vi "Simple Serial.vi"() -> ()   [LabVIEW 2018]
doc: "This example performs a serial port write and a serial port read. The parameters set for the serial port must match the parameters of the connected instrument or device. The VISA Configure Serial Port VI sets the configuration parameters. The front panel displays the controls used to configure the basic parameters, such as baud rate, data bits, and parity. The VI passes the VISA resource name to other VIs that perform operations on that VISA resource. The VISA Write function sends a command to the serial device and the VISA Read function returns data based on the command. The VISA Close function then closes the reference to the serial device. It is important to close the reference; otherwise, further communication through that port might not be possible."
uses:
  <vilib>/Instr/_visa.llb/VISA Configure Serial Port (Instr).vi
  <vilib>/Utility/file.llb/Write Delimited Spreadsheet (string).vi
panel:
  in  "ok":bool
  out "File Path Control":path
  in  "Select Sensor":bool[](array[boolean])
  out "Sensor In Graph":dbl
  in  "stop":bool
  out "chart":T1(graph)
  in  "?":string[][](table)
  in  "Serial Settings":T2={"Number of sen"=0.0, "Baud rate"=9600, "Separator"="", "COM"="COM1"} {"Baud rate" items=["75"=75, "110"=110, "134"=134, "150"=150, "300"=300, "600"=600, "1200"=1200, "1800"=1800, "2400"=2400, "4800"=4800, "7200"=7200, "9600"=9600, "14400"=14400, "19200"=19200, "28800"=28800, "38400"=38400, "56000"=56000, "57600"=57600, "115200"=115200, "128000"=128000, "230400"=230400]}
  in  "Clear":bool
  out "working sensor indexes 2":i32[](array[numeric])
  out "Counter":dbl
  out "working sensor index":dbl[](array[numeric])
  out "working sensor":dbl[](array[numeric])
  out "output array":dbl[](array[numeric])
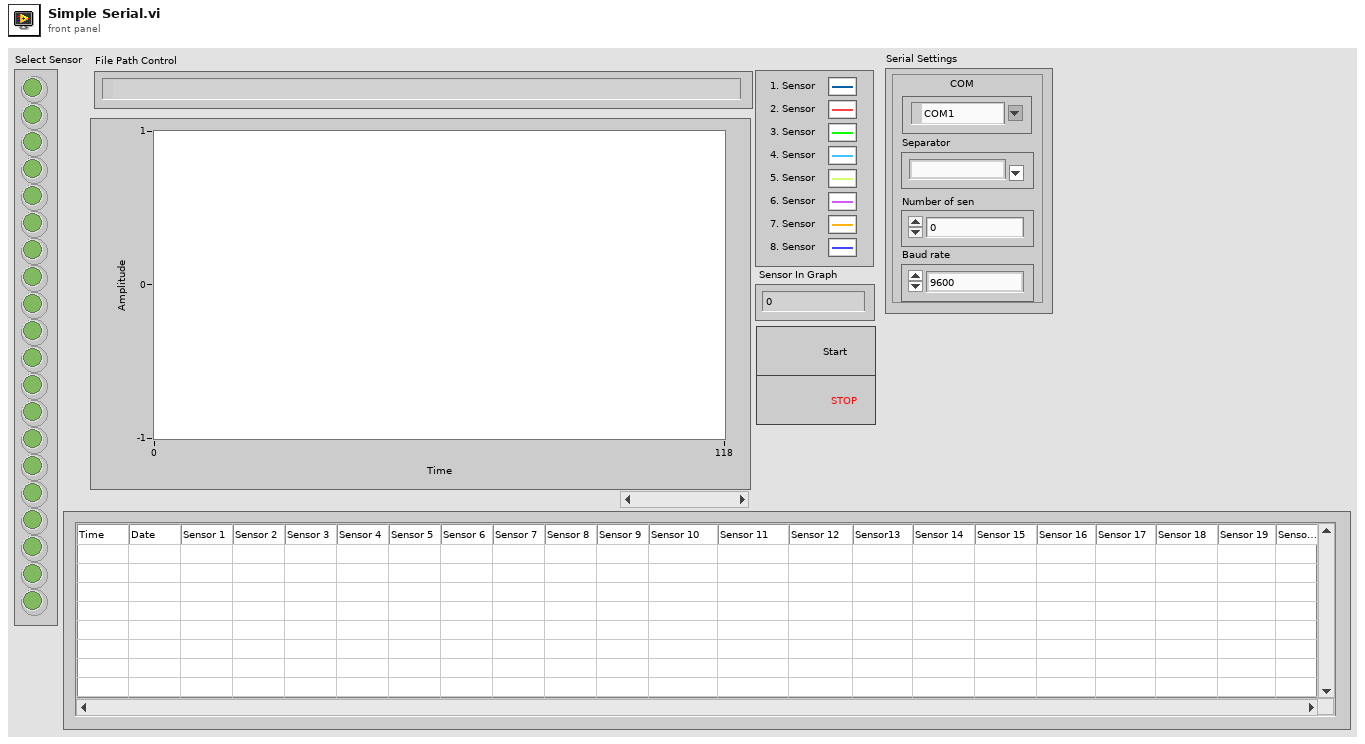
[diagram p1: front panel]
types:
  T1 = cluster{"element":dbl, "element":dbl, "element":dbl, "element":dbl, "element":dbl, "element":dbl, "element":dbl, "element":dbl}
  T2 = cluster{"Number of sen":dbl, "Baud rate":u32, "Separator":string, "COM":refnum<visa-resource-name>}
  T3 = cluster{"element":dbl, "element":dbl, "element":dbl, "element":dbl, "element":dbl, "element":dbl, "element":dbl, "element":dbl}[]
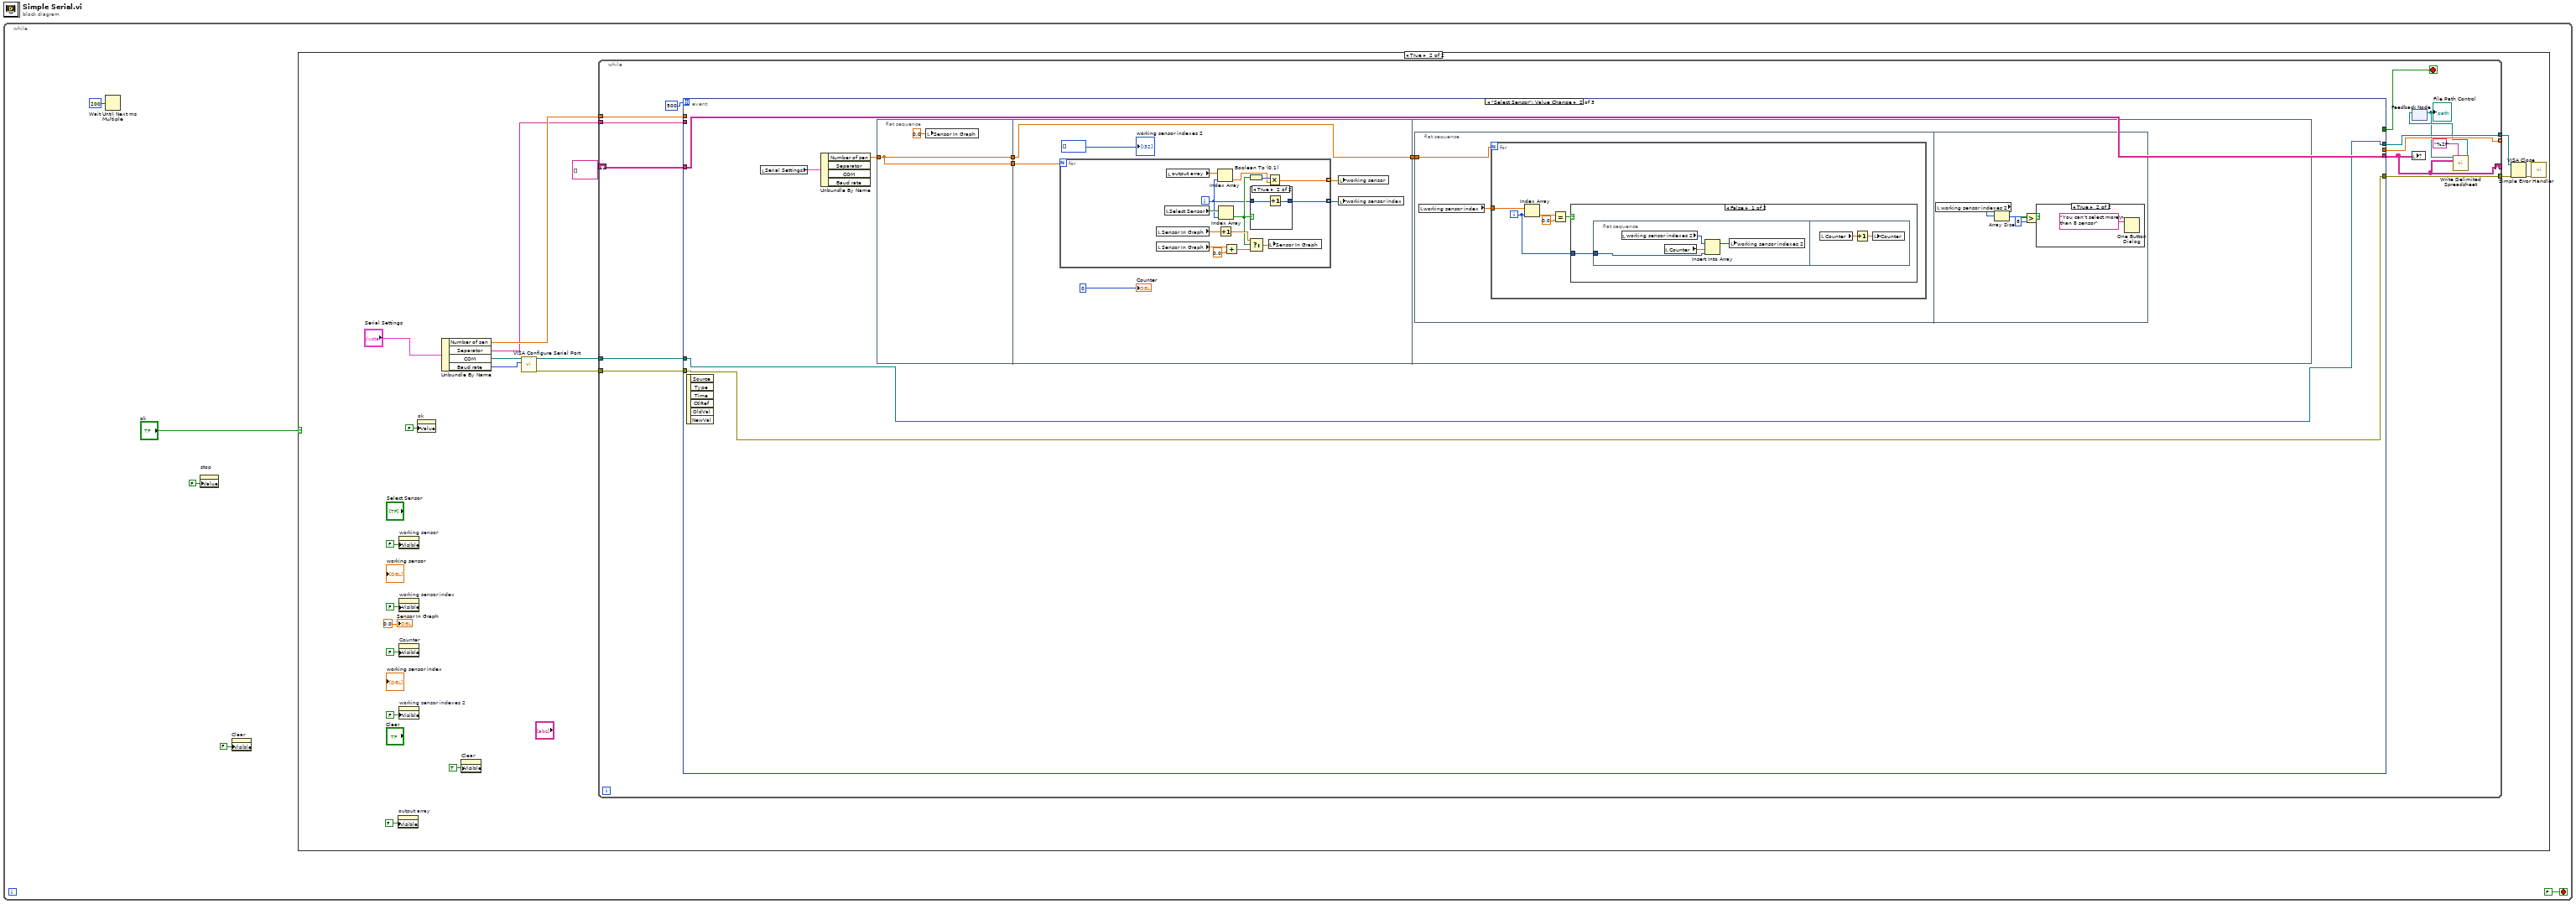
[diagram p0: block diagram]
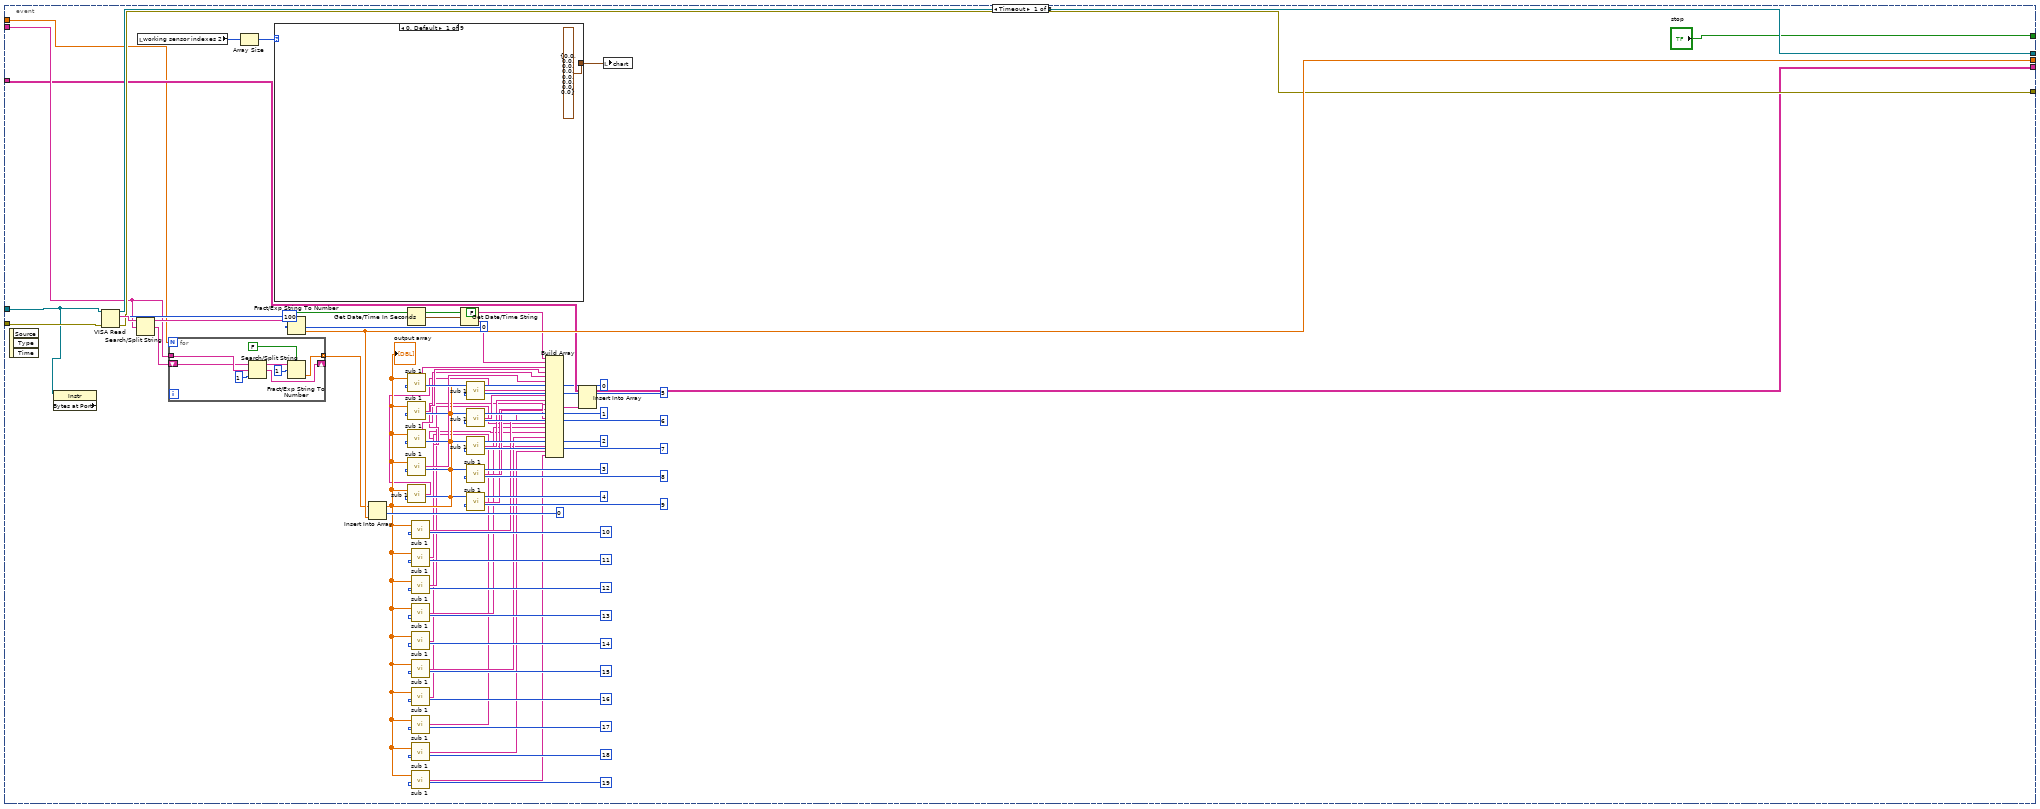
[diagram p3: hidden frame]
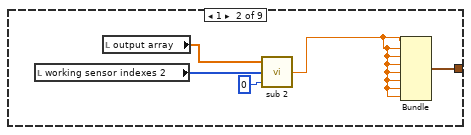
[diagram p4: hidden frame]
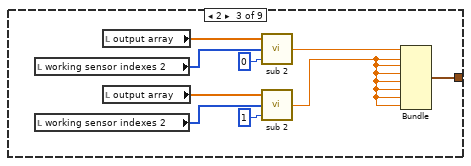
[diagram p5: hidden frame]
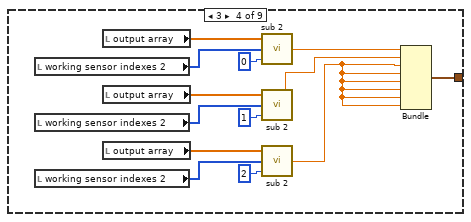
[diagram p6: hidden frame]
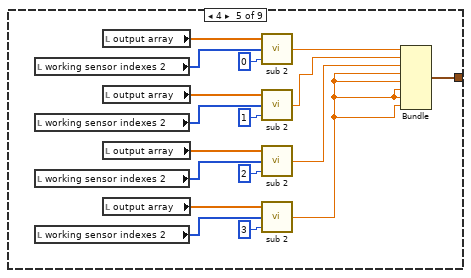
[diagram p7: hidden frame]
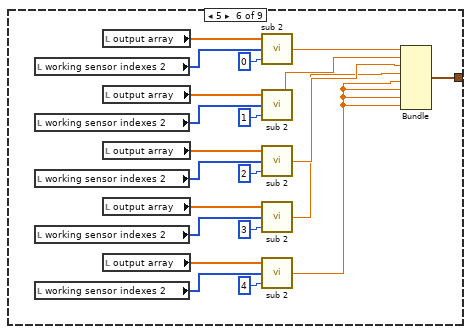
[diagram p8: hidden frame]
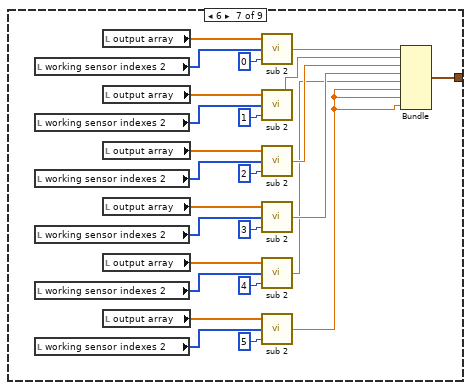
[diagram p9: hidden frame]
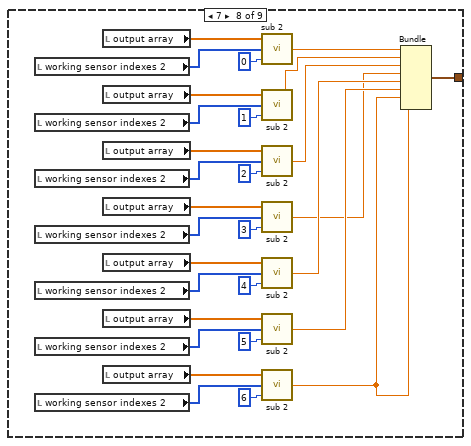
[diagram p10: hidden frame]
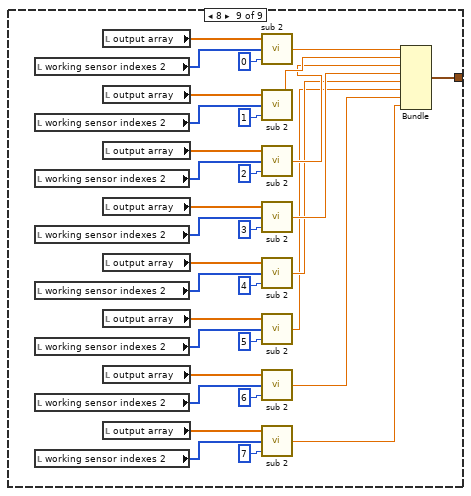
[diagram p11: hidden frame]
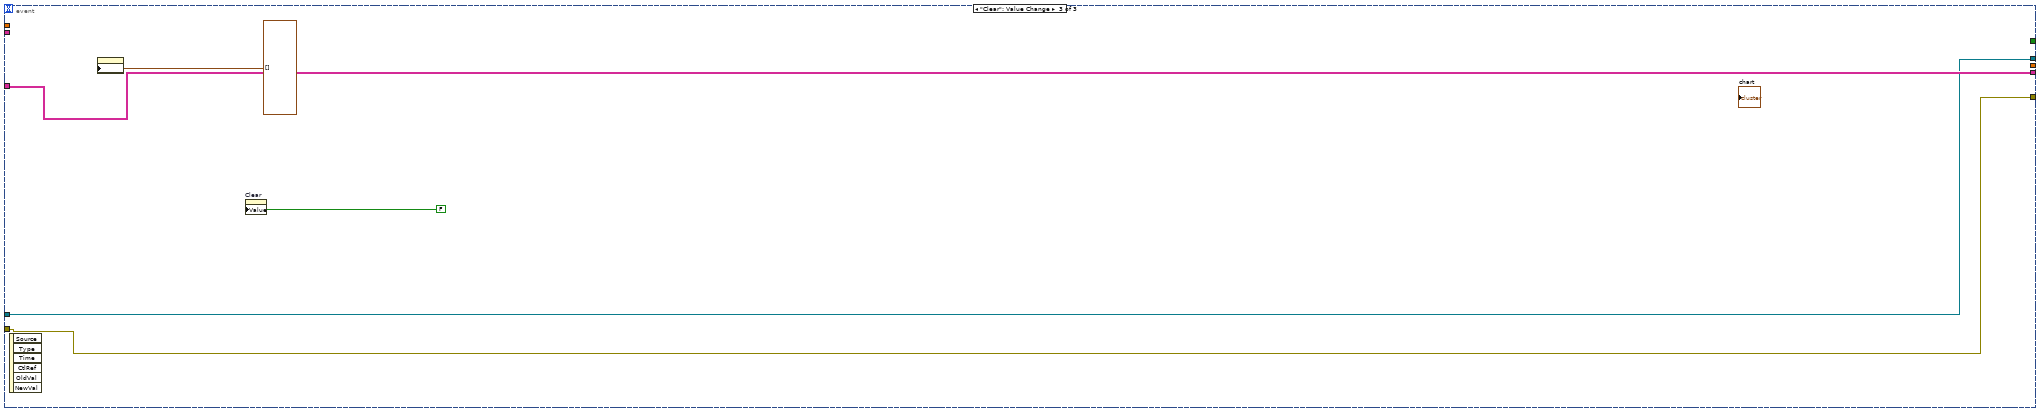
[diagram p15: hidden frame]
diagram:
  n1 = while {
    stop <- FALSE stop-if-true
    n2 = Wait Until Next ms Multiple(millisecond multiple=u32 200) -> ()  [unwired: 1 out]
    n3 = property on="stop" class="Bool (strict)"("Value"=FALSE) -> ()  [unwired: 2 in, 2 out]
    n4 = property on="Clear" class="Bool (strict)"("Visible"=FALSE) -> ()  [unwired: 2 in, 2 out]
    n5 = case shown="True" "ok" {
      frame False {
      }
      frame True {
        n6 = property on="output array" class="Arr (strict)"("Visible"=FALSE) -> ()  [unwired: 2 in, 2 out]
        n7 = property on="working sensor" class="Arr (strict)"("Visible"=FALSE) -> ()  [unwired: 2 in, 2 out]
        n8 = property on="working sensor index" class="Arr (strict)"("Visible"=FALSE) -> ()  [unwired: 2 in, 2 out]
        n9 = property on="Counter" class="DigNum (strict)"("Visible"=FALSE) -> ()  [unwired: 2 in, 2 out]
        n10 = property on="working sensor indexes 2" class="Arr (strict)"("Visible"=FALSE) -> ()  [unwired: 2 in, 2 out]
        n11 = property on="ok" class="Bool (strict)"("Value"=FALSE ("ok")) -> ()  [unwired: 2 in, 2 out]
        n12 = Unbundle By Name("Serial Settings") -> ("Number of sen"=w17:dbl, "Separator"=w16:string, "COM"=w18:refnum<visa-resource-name>, "Baud rate"=w19:u32)
        n13 = property on="Clear" class="Bool (strict)"("Visible"=TRUE) -> ()  [unwired: 2 in, 2 out]
        n14 = call-poly "VISA Configure Serial Port"("VISA resource name"=w18, "baud rate (9600)"=w19) -> ("VISA resource name out"=w7:refnum<visa-resource-name>, "error out"=w21:errorcluster)  [unwired: 7 in, 5 out]
        n15 = while {
          tunnel: w7 -> [w38]
          tunnel: [w33] -> w23
          tunnel: w21 -> [w37]
          tunnel: [w34] -> w24
          tunnel: [w35] -> _ mode=indexing
          tunnel: w17 -> [w36]
          tunnel: w16 -> [w31]
          shift-right: [w28] -> _
          shift-left: string[][] [] -> [w30]
          stop <- w25 stop-if-true
          n16 = event shown="[1] \"Select Sensor\": Value Change" {
            selector: _ -> [_ _ _]
            dyn-events: _ -> [_ _ _]
            timeout: 500 -> [_ _ _]
            tunnel: w38 -> [w41 w267 w319]
            tunnel: w37 -> [w104 w266 w318]
            tunnel: w36 -> [w45 _ _]
            tunnel: [w103 _ _] -> w35
            tunnel: [w96 w266 w318] -> w34
            tunnel: [w95 w267 w319] -> w33
            tunnel: w31 -> [w94 _ _]
            tunnel: [w88 w268 w322] -> w28
            tunnel: w30 -> [w93 w268 w322]
            tunnel: ["stop" _ _] -> w25
            event Timeout {
              n17 = event-data() -> ()  [unwired: 1 in, 3 out]
              n18 = property on="Property Node" class="Instr" props=["Bytes at Port"](reference=w41) -> ()  [unwired: 1 in, 3 out]
              n19 = VISA Read(VISA resource name=w41, byte count=u32 100, error in (no error)=w104) -> (VISA resource name out=w95:refnum<visa-resource-name>, read buffer=w100:string, error out=w96:errorcluster)  [unwired: 1 out]
              n20 = Search/Split String(string=w100, search string/char (-)=w94) -> (substring before match=w101:string, match + rest of string=w102:string)  [unwired: 1 in, 1 out]
              n21 = local read "working sensor indexes 2"() -> (w44:i32[])
              n22 = for {
                N: w45 -> [_]
                tunnel: w94 -> [w264]
                shift-right: [w259] -> _
                shift-left: w102 -> [w263]
                tunnel: [w261] -> w87 mode=indexing
                n23 = Search/Split String(string=w263, search string/char (-)=w264, offset (0)=1) -> (substring before match=w260:string, match + rest of string=w259:string)  [unwired: 1 out]
                n24 = Fract/Exp String To Number(use system decimal point (T)=FALSE, string=w260, offset=1) -> (number=w261:dbl)  [unwired: 1 in, 1 out]
              }
              n25 = Array Size(array=w44) -> (size(s)=w43:i32)
              n26 = case shown="0, Default" w43 {
                tunnel: [T1 {"element"=0.0, "element"=0.0, "element"=0.0, "element"=0.0, "element"=0.0, "element"=0.0, "element"=0.0, "element"=0.0} w106 w112 w123 w133 w150 w171 w198 w229] -> w42
                frame 0, Default {
                }
                frame 1 {
                  n27 = local read "working sensor indexes 2"() -> (w109:i32[])
                  n28 = local read "output array"() -> (w110:dbl[])
                  n29 = call "sub 2.vi"("index"=0, "array 2"=w109, "array"=w110) -> ("element"=w107:dbl)
                  n30 = Bundle("element"=w107, "element"=w107, "element"=w107, "element"=w107, "element"=w107, "element"=w107, "element"=w107, "element"=w107) -> (w106:T1)  [unwired: 1 in]
                }
                frame 2 {
                  n31 = local read "working sensor indexes 2"() -> (w115:i32[])
                  n32 = local read "working sensor indexes 2"() -> (w118:i32[])
                  n33 = local read "output array"() -> (w114:dbl[])
                  n34 = local read "output array"() -> (w119:dbl[])
                  n35 = call "sub 2.vi"("index"=0, "array 2"=w115, "array"=w114) -> ("element"=w113:dbl)
                  n36 = call "sub 2.vi"("index"=1, "array 2"=w118, "array"=w119) -> ("element"=w111:dbl)
                  n37 = Bundle("element"=w113, "element"=w111, "element"=w111, "element"=w111, "element"=w111, "element"=w111, "element"=w111, "element"=w111) -> (w112:T1)  [unwired: 1 in]
                }
                frame 3 {
                  n38 = local read "working sensor indexes 2"() -> (w131:i32[])
                  n39 = local read "working sensor indexes 2"() -> (w130:i32[])
                  n40 = local read "working sensor indexes 2"() -> (w124:i32[])
                  n41 = local read "output array"() -> (w132:dbl[])
                  n42 = local read "output array"() -> (w129:dbl[])
                  n43 = local read "output array"() -> (w125:dbl[])
                  n44 = call "sub 2.vi"("index"=0, "array 2"=w131, "array"=w132) -> ("element"=w122:dbl)
                  n45 = call "sub 2.vi"("index"=1, "array 2"=w130, "array"=w129) -> ("element"=w121:dbl)
                  n46 = call "sub 2.vi"("index"=2, "array 2"=w124, "array"=w125) -> ("element"=w120:dbl)
                  n47 = Bundle("element"=w122, "element"=w121, "element"=w120, "element"=w120, "element"=w120, "element"=w120, "element"=w120, "element"=w120) -> (w123:T1)  [unwired: 1 in]
                }
                frame 4 {
                  n48 = local read "working sensor indexes 2"() -> (w148:i32[])
                  n49 = local read "working sensor indexes 2"() -> (w149:i32[])
                  n50 = local read "working sensor indexes 2"() -> (w145:i32[])
                  n51 = local read "working sensor indexes 2"() -> (w140:i32[])
                  n52 = local read "output array"() -> (w147:dbl[])
                  n53 = local read "output array"() -> (w138:dbl[])
                  n54 = local read "output array"() -> (w146:dbl[])
                  n55 = local read "output array"() -> (w139:dbl[])
                  n56 = call "sub 2.vi"("index"=0, "array 2"=w148, "array"=w147) -> ("element"=w137:dbl)
                  n57 = call "sub 2.vi"("index"=1, "array 2"=w149, "array"=w138) -> ("element"=w136:dbl)
                  n58 = call "sub 2.vi"("index"=2, "array 2"=w145, "array"=w146) -> ("element"=w135:dbl)
                  n59 = call "sub 2.vi"("index"=3, "array 2"=w140, "array"=w139) -> ("element"=w134:dbl)
                  n60 = Bundle("element"=w137, "element"=w136, "element"=w135, "element"=w134, "element"=w134, "element"=w134, "element"=w134, "element"=w134) -> (w133:T1)  [unwired: 1 in]
                }
                frame 5 {
                  n61 = local read "working sensor indexes 2"() -> (w170:i32[])
                  n62 = local read "working sensor indexes 2"() -> (w169:i32[])
                  n63 = local read "working sensor indexes 2"() -> (w166:i32[])
                  n64 = local read "working sensor indexes 2"() -> (w165:i32[])
                  n65 = local read "working sensor indexes 2"() -> (w157:i32[])
                  n66 = local read "output array"() -> (w156:dbl[])
                  n67 = local read "output array"() -> (w168:dbl[])
                  n68 = local read "output array"() -> (w167:dbl[])
                  n69 = local read "output array"() -> (w164:dbl[])
                  n70 = local read "output array"() -> (w158:dbl[])
                  n71 = call "sub 2.vi"("index"=0, "array 2"=w170, "array"=w156) -> ("element"=w155:dbl)
                  n72 = call "sub 2.vi"("index"=1, "array 2"=w169, "array"=w168) -> ("element"=w154:dbl)
                  n73 = call "sub 2.vi"("index"=2, "array 2"=w166, "array"=w167) -> ("element"=w153:dbl)
                  n74 = call "sub 2.vi"("index"=3, "array 2"=w165, "array"=w164) -> ("element"=w152:dbl)
                  n75 = call "sub 2.vi"("index"=4, "array 2"=w157, "array"=w158) -> ("element"=w151:dbl)
                  n76 = Bundle("element"=w155, "element"=w154, "element"=w153, "element"=w152, "element"=w151, "element"=w151, "element"=w151, "element"=w151) -> (w150:T1)  [unwired: 1 in]
                }
                frame 6 {
                  n77 = local read "working sensor indexes 2"() -> (w195:i32[])
                  n78 = local read "working sensor indexes 2"() -> (w194:i32[])
                  n79 = local read "working sensor indexes 2"() -> (w191:i32[])
                  n80 = local read "working sensor indexes 2"() -> (w190:i32[])
                  n81 = local read "working sensor indexes 2"() -> (w182:i32[])
                  n82 = local read "working sensor indexes 2"() -> (w181:i32[])
                  n83 = local read "output array"() -> (w178:dbl[])
                  n84 = local read "output array"() -> (w193:dbl[])
                  n85 = local read "output array"() -> (w192:dbl[])
                  n86 = local read "output array"() -> (w189:dbl[])
                  n87 = local read "output array"() -> (w183:dbl[])
                  n88 = local read "output array"() -> (w180:dbl[])
                  n89 = call "sub 2.vi"("index"=0, "array 2"=w195, "array"=w178) -> ("element"=w177:dbl)
                  n90 = call "sub 2.vi"("index"=1, "array 2"=w194, "array"=w193) -> ("element"=w176:dbl)
                  n91 = call "sub 2.vi"("index"=2, "array 2"=w191, "array"=w192) -> ("element"=w175:dbl)
                  n92 = call "sub 2.vi"("index"=3, "array 2"=w190, "array"=w189) -> ("element"=w174:dbl)
                  n93 = call "sub 2.vi"("index"=4, "array 2"=w182, "array"=w183) -> ("element"=w173:dbl)
                  n94 = call "sub 2.vi"("index"=5, "array 2"=w181, "array"=w180) -> ("element"=w172:dbl)
                  n95 = Bundle("element"=w177, "element"=w176, "element"=w175, "element"=w174, "element"=w173, "element"=w172, "element"=w172, "element"=w172) -> (w171:T1)  [unwired: 1 in]
                }
                frame 7 {
                  n96 = local read "working sensor indexes 2"() -> (w224:i32[])
                  n97 = local read "working sensor indexes 2"() -> (w223:i32[])
                  n98 = local read "working sensor indexes 2"() -> (w220:i32[])
                  n99 = local read "working sensor indexes 2"() -> (w219:i32[])
                  n100 = local read "working sensor indexes 2"() -> (w206:i32[])
                  n101 = local read "working sensor indexes 2"() -> (w207:i32[])
                  n102 = local read "working sensor indexes 2"() -> (w210:i32[])
                  n103 = local read "output array"() -> (w205:dbl[])
                  n104 = local read "output array"() -> (w222:dbl[])
                  n105 = local read "output array"() -> (w221:dbl[])
                  n106 = local read "output array"() -> (w218:dbl[])
                  n107 = local read "output array"() -> (w200:dbl[])
                  n108 = local read "output array"() -> (w208:dbl[])
                  n109 = local read "output array"() -> (w209:dbl[])
                  n110 = call "sub 2.vi"("index"=0, "array 2"=w224, "array"=w205) -> ("element"=w204:dbl)
                  n111 = call "sub 2.vi"("index"=1, "array 2"=w223, "array"=w222) -> ("element"=w203:dbl)
                  n112 = call "sub 2.vi"("index"=2, "array 2"=w220, "array"=w221) -> ("element"=w202:dbl)
                  n113 = call "sub 2.vi"("index"=3, "array 2"=w219, "array"=w218) -> ("element"=w197:dbl)
                  n114 = call "sub 2.vi"("index"=4, "array 2"=w206, "array"=w200) -> ("element"=w201:dbl)
                  n115 = call "sub 2.vi"("index"=5, "array 2"=w207, "array"=w208) -> ("element"=w199:dbl)
                  n116 = call "sub 2.vi"("index"=6, "array 2"=w210, "array"=w209) -> ("element"=w196:dbl)
                  n117 = Bundle("element"=w204, "element"=w203, "element"=w202, "element"=w197, "element"=w201, "element"=w199, "element"=w196, "element"=w196) -> (w198:T1)  [unwired: 1 in]
                }
                frame 8 {
                  n118 = local read "working sensor indexes 2"() -> (w257:i32[])
                  n119 = local read "working sensor indexes 2"() -> (w256:i32[])
                  n120 = local read "working sensor indexes 2"() -> (w253:i32[])
                  n121 = local read "working sensor indexes 2"() -> (w252:i32[])
                  n122 = local read "working sensor indexes 2"() -> (w246:i32[])
                  n123 = local read "working sensor indexes 2"() -> (w247:i32[])
                  n124 = local read "working sensor indexes 2"() -> (w250:i32[])
                  n125 = local read "working sensor indexes 2"() -> (w226:i32[])
                  n126 = local read "output array"() -> (w245:dbl[])
                  n127 = local read "output array"() -> (w255:dbl[])
                  n128 = local read "output array"() -> (w254:dbl[])
                  n129 = local read "output array"() -> (w251:dbl[])
                  n130 = local read "output array"() -> (w239:dbl[])
                  n131 = local read "output array"() -> (w248:dbl[])
                  n132 = local read "output array"() -> (w249:dbl[])
                  n133 = local read "output array"() -> (w227:dbl[])
                  n134 = call "sub 2.vi"("index"=0, "array 2"=w257, "array"=w245) -> ("element"=w244:dbl)
                  n135 = call "sub 2.vi"("index"=1, "array 2"=w256, "array"=w255) -> ("element"=w243:dbl)
                  n136 = call "sub 2.vi"("index"=2, "array 2"=w253, "array"=w254) -> ("element"=w242:dbl)
                  n137 = call "sub 2.vi"("index"=3, "array 2"=w252, "array"=w251) -> ("element"=w241:dbl)
                  n138 = call "sub 2.vi"("index"=4, "array 2"=w246, "array"=w239) -> ("element"=w240:dbl)
                  n139 = call "sub 2.vi"("index"=5, "array 2"=w247, "array"=w248) -> ("element"=w238:dbl)
                  n140 = call "sub 2.vi"("index"=6, "array 2"=w250, "array"=w249) -> ("element"=w237:dbl)
                  n141 = call "sub 2.vi"("index"=7, "array 2"=w226, "array"=w227) -> ("element"=w225:dbl)
                  n142 = Bundle("element"=w244, "element"=w243, "element"=w242, "element"=w241, "element"=w240, "element"=w238, "element"=w237, "element"=w225) -> (w229:T1)  [unwired: 1 in]
                }
              }
              n143 = Fract/Exp String To Number(use system decimal point (T)=FALSE, string=w101, offset=0) -> (number=w103:dbl)  [unwired: 1 in, 1 out]
              n144 = Insert Into Array(array=w87, index=0, new element=w103) -> (w66:dbl[])
              "output array" <- w66
              n145 = Get Date/Time In Seconds() -> (seconds since 1Jan1904=w92:timestamp)
              n146 = call "sub 1.vi"("index"=0, "array"=w66) -> ("resulting string"=w65:string)
              n147 = call "sub 1.vi"("index"=1, "array"=w66) -> ("resulting string"=w64:string)
              n148 = call "sub 1.vi"("index"=2, "array"=w66) -> ("resulting string"=w63:string)
              n149 = call "sub 1.vi"("index"=3, "array"=w66) -> ("resulting string"=w62:string)
              n150 = call "sub 1.vi"("index"=4, "array"=w66) -> ("resulting string"=w61:string)
              n151 = call "sub 1.vi"("index"=10, "array"=w66) -> ("resulting string"=w55:string)
              n152 = call "sub 1.vi"("index"=11, "array"=w66) -> ("resulting string"=w54:string)
              n153 = call "sub 1.vi"("index"=12, "array"=w66) -> ("resulting string"=w53:string)
              n154 = call "sub 1.vi"("index"=13, "array"=w66) -> ("resulting string"=w52:string)
              n155 = call "sub 1.vi"("index"=14, "array"=w66) -> ("resulting string"=w51:string)
              n156 = call "sub 1.vi"("index"=15, "array"=w66) -> ("resulting string"=w50:string)
              n157 = call "sub 1.vi"("index"=16, "array"=w66) -> ("resulting string"=w49:string)
              n158 = call "sub 1.vi"("index"=17, "array"=w66) -> ("resulting string"=w48:string)
              n159 = call "sub 1.vi"("index"=18, "array"=w66) -> ("resulting string"=w47:string)
              n160 = call "sub 1.vi"("index"=19, "array"=w66) -> ("resulting string"=w46:string)
              n161 = Get Date/Time String(seconds (now)=w92) -> (date string=w91:string, time string=w90:string)  [unwired: 2 in]
              n162 = call "sub 1.vi"("index"=5, "array"=w66) -> ("resulting string"=w60:string)
              n163 = call "sub 1.vi"("index"=6, "array"=w66) -> ("resulting string"=w59:string)
              n164 = call "sub 1.vi"("index"=7, "array"=w66) -> ("resulting string"=w58:string)
              n165 = call "sub 1.vi"("index"=8, "array"=w66) -> ("resulting string"=w57:string)
              n166 = call "sub 1.vi"("index"=9, "array"=w66) -> ("resulting string"=w56:string)
              n167 = Build Array(w91, w90, w65, w64, w63, w62, w61, w60, w59, w58, w57, w56, w55, w54, w53, w52, w51, w50, w49, w48, w47, w46) -> (w89:string[])
              n168 = Insert Into Array(array=w93, new element=w89) -> (w88:string[][])  [unwired: 2 in]
              n169 = local write "chart"(w42) -> ()
            }
            event "Select Sensor": Value Change {
              n170 = event-data() -> ()  [unwired: 1 in, 6 out]
              n171 = local read "Serial Settings"() -> (w273:T2)
              n172 = Unbundle By Name(w273) -> ("Number of sen"=w272:dbl)  [unwired: 3 out]
              n173 = flat-sequence {
                tunnel: w272 -> [w274]
                tunnel: [w274] -> w271
                tunnel: [w274] -> w269
                tunnel: w271 -> [w281]
                tunnel: [w278] -> w270
                tunnel: w269 -> [w278]
                tunnel: w270 -> [w298]
                frame #0 {
                  n174 = local write "Sensor In Graph"(0.0 ("y")) -> ()
                }
                frame #1 {
                  n175 = for {
                    N: w281 -> [_]
                    tunnel: [w291] -> w280 mode=indexing
                    tunnel: [w282] -> w279 mode=indexing
                    i -> [w283]
                    n176 = local read "Sensor In Graph"() -> (w286:dbl)
                    n177 = local read "Sensor In Graph"() -> (w290:dbl)
                    n178 = local read "Select Sensor"() -> (w295:bool[])
                    n179 = local read "output array"() -> (w294:dbl[])
                    n180 = Index Array(array=w294, index=w283) -> (element=w292:dbl)
                    n181 = Increment(x=w286) -> (x+1=w287:dbl)
                    n182 = Index Array(array=w295, index=w283) -> (element=w284:bool)
                    n183 = Add(x=w290, y=0.0) -> (x+y=w288:dbl)
                    n184 = Boolean To (0,1)(Boolean=w284) -> (0, 1=w293:i16)
                    n185 = Select(t=w287, s=w284, f=w288) -> (s? t:f=w285:dbl)
                    n186 = case shown="True" w284 {
                      tunnel: w283 -> [_ w297]
                      tunnel: [_ w296] -> w282
                      frame False {
                      }
                      frame True {
                        n187 = Increment(x=w297) -> (x+1=w296:i32)
                      }
                    }
                    n188 = Multiply(x=w293, y=w292) -> (x*y=w291:dbl)
                    n189 = local write "Sensor In Graph"(w285) -> ()
                  }
                  n190 = local write "working sensor"(w280) -> ()
                  n191 = local write "working sensor index"(w279) -> ()
                  "Counter" <- 0 ("index")
                  "working sensor indexes 2" <- i32[] [] ("array")
                }
                frame #2 {
                  n192 = flat-sequence {
                    tunnel: w298 -> [w300]
                    frame #0 {
                      n193 = local read "working sensor index"() -> (w299:dbl[])
                      n194 = for {
                        N: w300 -> [_]
                        tunnel: w299 -> [w302]
                        i -> [w301]
                        n195 = Index Array(array=w302, index=w301) -> (element=w303:dbl)
                        n196 = Equal?(x=w303, y=0.0) -> (x = y?=w305:bool)
                        n197 = case shown="False" w305 {
                          tunnel: w301 -> [w306 _]
                          frame False {
                            n198 = flat-sequence {
                              tunnel: w306 -> [w307]
                              frame #0 {
                                n199 = local read "working sensor indexes 2"() -> (w308:i32[])
                                n200 = local read "Counter"() -> (w310:dbl)
                                n201 = Insert Into Array(array=w308, index=w310, new element=w307) -> (w309:i32[])
                                n202 = local write "working sensor indexes 2"(w309) -> ()
                              }
                              frame #1 {
                                n203 = local read "Counter"() -> (w311:dbl)
                                n204 = Increment(x=w311) -> (x+1=w312:dbl)
                                n205 = local write "Counter"(w312) -> ()
                              }
                            }
                          }
                          frame True {
                          }
                        }
                      }
                    }
                    frame #1 {
                      n206 = local read "working sensor indexes 2"() -> (w315:i32[])
                      n207 = Array Size(array=w315) -> (size(s)=w314:i32)
                      n208 = Greater?(x=w314, y=8) -> (0:w316:bool)
                      n209 = case shown="True" w316 {
                        frame False {
                        }
                        frame True {
                          n210 = One Button Dialog(message="You can't select more\n than 8 sensor") -> ()  [unwired: 1 in, 1 out]
                        }
                      }
                    }
                  }
                }
              }
            }
            event "Clear": Value Change {
              n211 = event-data() -> ()  [unwired: 1 in, 6 out]
              n212 = property on="chart" class="WFChart (strict)"("History Data"=T3 []) -> ()  [unwired: 2 in, 2 out]
              n213 = property on="Clear" class="Bool (strict)"("Value"=FALSE ("Visible")) -> ()  [unwired: 2 in, 2 out]
            }
          }
          n214 = feedback #1() -> (w26:path)  [unwired: 1 in]
          "File Path Control" <- w26
          n215 = local write item#3(w28) -> ()
          n216 = call-poly <vilib>:"Write Delimited Spreadsheet.vi"("file path (dialog if empty)"=w26, "format (%s)"="%2f" ("format string"), "2D data"=w28) -> ("new file path (Not A Path if cancelled)"=w27:path)  [unwired: 11 in, 1 out]
          n217 = feedback-in #1(w27) -> ()
        }
        n218 = VISA Close(VISA resource name=w23, error in (no error)=w24) -> (error out=w22:errorcluster)
        n219 = call <vilib>:"Simple Error Handler.vi"("error in (no error)"=w22) -> ()  [unwired: 1 in, 8 out]
        "Sensor In Graph" <- 0.0 ("Number  Sensor")
      }
    }
  }
